vi "RT_Controller.vi"() -> ()   [LabVIEW 2017]
doc: "RT Controller with the coordinate transformation implemented, and with DSA!\n\nfor controlling FPGA controller with feedback linearization"
uses:
  <vilib>/rvi/interface/nirviReadWriteControl/nirviReadWriteControl.xnode
  <vilib>/Platform/TimedLoop/XDataNode/XDataNode.xnode
  <vilib>/Platform/TimedLoop/XDataNode/nitl_modes.ctl
  <vilib>/Platform/TimedLoop/XDataNode/XDNodeRunTimeDep.lvlib
  <vilib>/Platform/TimedLoop/XDataNode/wakeup.ctl
  <vilib>/Platform/TimedLoop/XDataNode/timing_clust.ctl
  Components/Timing/Timing.lvlib
  <vilib>/rvi/interface/nirviOpenFPGA/nirviOpenFPGA.xnode
  <vilib>/NI/STM/NI STM.lvlib
  <vilib>/NI/STM/SubVIs/MetaDataElement.ctl
  <vilib>/rvi/interface/nirviCloseFPGA/nirviCloseFPGA.xnode
  Components/DSA/DSA.lvlib
  <vilib>/Analysis/NI_AALPro.lvlib
  <vilib>/NI/STM/TCP/Write Message (TCP).vi
  TypeDefs/FPGA VI Reference.ctl
  <vilib>/ptbypt/NI_PtbyPt.lvlib
  TypeDefs/Ki.ctl
  <vilib>/NI/STM/TCP/Get Connection Reference (TCP).vi
  <vilib>/NI/STM/TCP/Write Meta Data (TCP Ref).vi
  FPGA Bitfiles/flexlab_FPGATarget_Tbeam256MAMainVI_XFHOL9u-69o.lvbitx
  NiFpgaLv.dll
  <vilib>/Utility/error.llb/Error Cluster From Error Code.vi
  <vilib>/rvi/errors/niLvFpgaAdjustHostInterfaceError.vi
  <vilib>/FPGAPlugInAG/myRIO-1900/niLvFpga_Close_myRIO-1900.vi
  <vilib>/FPGAPlugInAG/myRIO-1900/niLvFpga_Open_myRIO-1900.vi
  Components/SignalGen/SignalGenParams_Cluster.ctl
  Components/SignalGen/SignalGen.lvlib
  TypeDefs/ChZero_Cluster.ctl
  TypeDefs/BendTwist_Ref_Cluster.ctl
  TypeDefs/Kp.ctl
  TypeDefs/RefChEnum.ctl
panel:
  in  "Timing":enum32{"RT Loop", "DSA Loop", "While Loop"}(tab)=enum."While Loop"
  out "Finished late?":dbl
  out "Loop rate [Hz]":dbl=2000.0 min=0.0 step=100.0 format="%.2p"
  out "Finished late?":dbl
  out "Loop rate [Hz]":dbl=2000.0 min=0.0 step=100.0 format="%.2p"
  out "Number of iterations":i32
  in  "Select Operation Mode":enum32{"Settings", "Closed Loop"}(tab)=enum."Closed Loop"
  in  "Reset Zero":bool
  in  "Set Measurement Zero":bool
  in  "ChZero_Cluster":T1={"Bend Zero [V]"=-2.668583393096924, "Twist Zero [V]"=-0.010879039764404297} {"Twist Zero [V]" step=0.1; "Bend Zero [V]" step=0.1}
  in  "Twist Lead":T3={"Twist Lead Num (a0,a1)"=[-0.144109583, 0.144363337, 120.0], "Twist Lead Den (b0,b1)"=[0.984133655, -1.983879901, 120.0]} {"Twist Lead Den (b0,b1)" format="%#_5e"; "Twist Lead Num (a0,a1)" format="%#_5e"}
  in  "Ref Ch.":T4
  in  "Ref_Cluster":T5 {"Twist_ref [V]" step=0.001; "Bend_ref [V]" min=0.0 step=0.005 format="%#.4f"}
  in  "Run \nController?":bool
  in  "Kp":T6=[25.0, 20.0, 100000.0] format="%#_6p"
  in  "Ki*Ts":T2=[0.00062, 0.00045, 120.0] format="%#_5e"
  in  "Reference offset":T7={"phase"=0.0, "amplitude"=0.0, "frequency"=0.0, "offset"=0.0, "Signal"=enum."DSA"} {"offset" format="%0.2f"; "frequency" format="%#.4f"; "amplitude" step=0.01 format="%#.4f"; "phase" format="%0.2f"}
  in  "Bend Lead":T8={"Bend Lead Num (a0,a1)"=[-0.408503893706518, 0.409017557515985, 120.0], "Bend Lead Den (b0,b1)"=[0.968209299629241, -1.967695635819774, 120.0]} {"Bend Lead Den (b0,b1)" format="%#_5e"; "Bend Lead Num (a0,a1)" format="%#_5e"}
  in  "stop":bool
  in  "DSA":enum32{"DSA Controls", "DSA Plots"}(tab)
  in  "DSA Freq. Resp. Meas.":T9(ring)=enum."RR_bend"
  out "DSA\nRunning?":bool
  in  "Stop DSA":bool
  in  "Start DSA":bool
  in  "DSA excitation specs":T10={"Initial Freq. [Hz]"=5.0, "Final Freq. [Hz]"=990.0, "# pts. in interval"=30, "Samping Time [s]"=0.0005, "Amplitude"=0.01, "Offset [V]"=0.0, "Freq Units (F: rad/s, T: Hz)"=TRUE}
  in  "Cycle Specs":T11={"Cycles To \nSettle (M)"=5, "Cycles To \nCalculate (N)"=20}
  out "Phase Bode Plot":cluster{dbl[], dbl[]}(graph)
  out "Magnitude Bode Plot":cluster{dbl[], dbl[]}(graph)
  # "Run the PC_Controller.vi to enable running of main loop and transfer of data!"
  # "Make sure to select the correct Ref. Ch. \ne.g. RR_Bend requires \nRef. Ch. to be Bend"
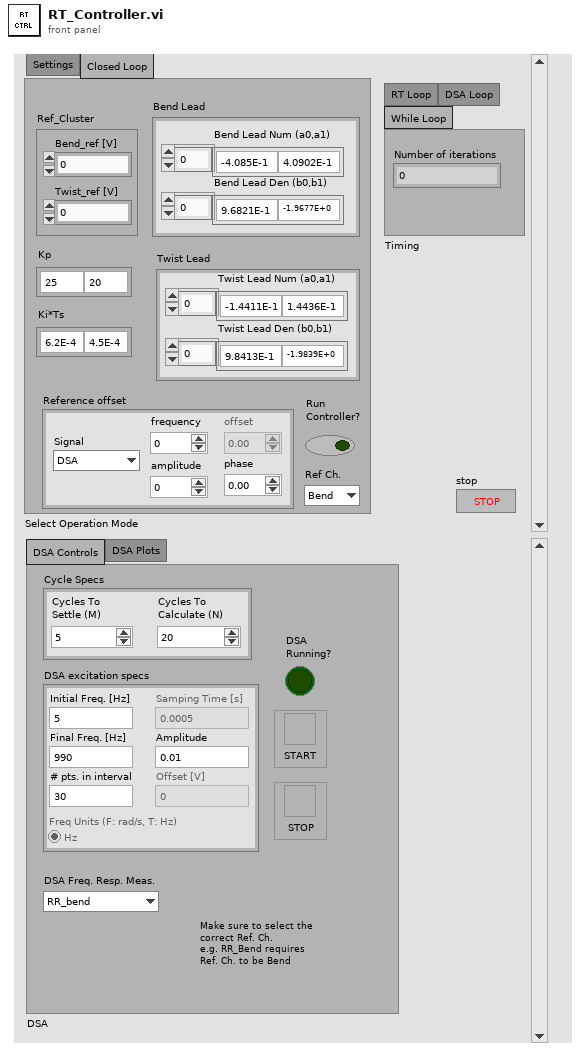
[diagram p1: front panel]
types:
  T1 = typedef "ChZero_Cluster.ctl" = cluster{"Bend Zero [V]":dbl, "Twist Zero [V]":dbl}
  T2 = typedef "Ki.ctl" = dbl[]
  T3 = cluster{"Twist Lead Num (a0,a1)":T2, "Twist Lead Den (b0,b1)":T2}
  T4 = typedef "RefChEnum.ctl" = enum16{"Bend", "Twist"}
  T5 = typedef "BendTwist_Ref_Cluster.ctl" = cluster{"Bend_ref [V]":dbl, "Twist_ref [V]":dbl}
  T6 = typedef "Kp.ctl" = dbl[]
  T7 = typedef "SignalGen.lvlib/SignalGenParams_Cluster.ctl" = cluster{"phase":dbl, "amplitude":dbl, "frequency":dbl, "offset":dbl, "Signal":enum16{"DC", "Sine", "Square", "Triangle", "Sawtooth", "DSA"}}
  T8 = cluster{"Bend Lead Num (a0,a1)":T2, "Bend Lead Den (b0,b1)":T2}
  T9 = enum16{"Plant_bend", "Plant_twist", "RR_bend", "RR_twist", "Ctrl_bend", "Ctrl_twist"}
  T10 = cluster{"Initial Freq. [Hz]":dbl, "Final Freq. [Hz]":dbl, "# pts. in interval":i16, "Samping Time [s]":dbl, "Amplitude":dbl, "Offset [V]":dbl, "Freq Units (F: rad/s, T: Hz)":bool}
  T11 = cluster{"Cycles To \nSettle (M)":i16, "Cycles To \nCalculate (N)":i16}
  T12 = typedef "NI STM.lvlib/MetaDataElement.ctl" = string
  T13 = typedef "FPGA VI Reference.ctl" = refnum<k20>
  T14 = typedef "NI STM.lvlib/TCP Connection Info.ctl" = cluster{"connection ID":refnum<k5>, "meta data":T12[]}
  T15 = typedef "XDNodeRunTimeDep.lvlib/timing_clust.ctl" = cluster{"Expected End [f-1]":u64, "Actual End [f-1]":u64, "Finished Late? [f-1]":bool, "Expected End [i-1]":u64, "Actual End [i-1]":u64, "Finished Late? [i-1]":bool, "Expected Start [i]":u64, "Actual Start [i]":u64, "Expected Start [f]":u64, "Actual Start [f]":u64, "Source Name":string, "Structure Name":string, "Period":i64, "Deadline":i64, "Offset":i64, "Start":i64, "Priority":i32, "Timeout":i32, "Mode":T16, "Wakeup Reason":T17, "Error":errorcluster, "Source Type":string, "Secondary Source Type":string, "Global End Time":u64, "Global Start Time":u64, "Frame Duration":u64, "Iteration Duration":u64, "Assigned CPU":i32, "I/O Scan Engine Mode":u32}
  T16 = typedef "XDNodeRunTimeDep.lvlib/nitl_modes.ctl" = enum32{"No Change", "Process missed periods, maintain original phase", "Discard missed periods, maintain original phase", "Process missed periods, ignore original phase", "Discard missed periods, ignore original phase"}
  T17 = typedef "XDNodeRunTimeDep.lvlib/wakeup.ctl" = enum32{"Normal", "Aborted", "Asynchronous wakeup", "Timing source error", "Timed loop error", "Timeout"}
  T18 = cluster{"Bend":cluster{"Notch Num (a0,a1,a2)":T2, "Notch Den (b0,b1)":T2}, "Twist":cluster{"Notch Num (a0,a1,a2)":T2, "Notch Den (b0,b1)":T2}}
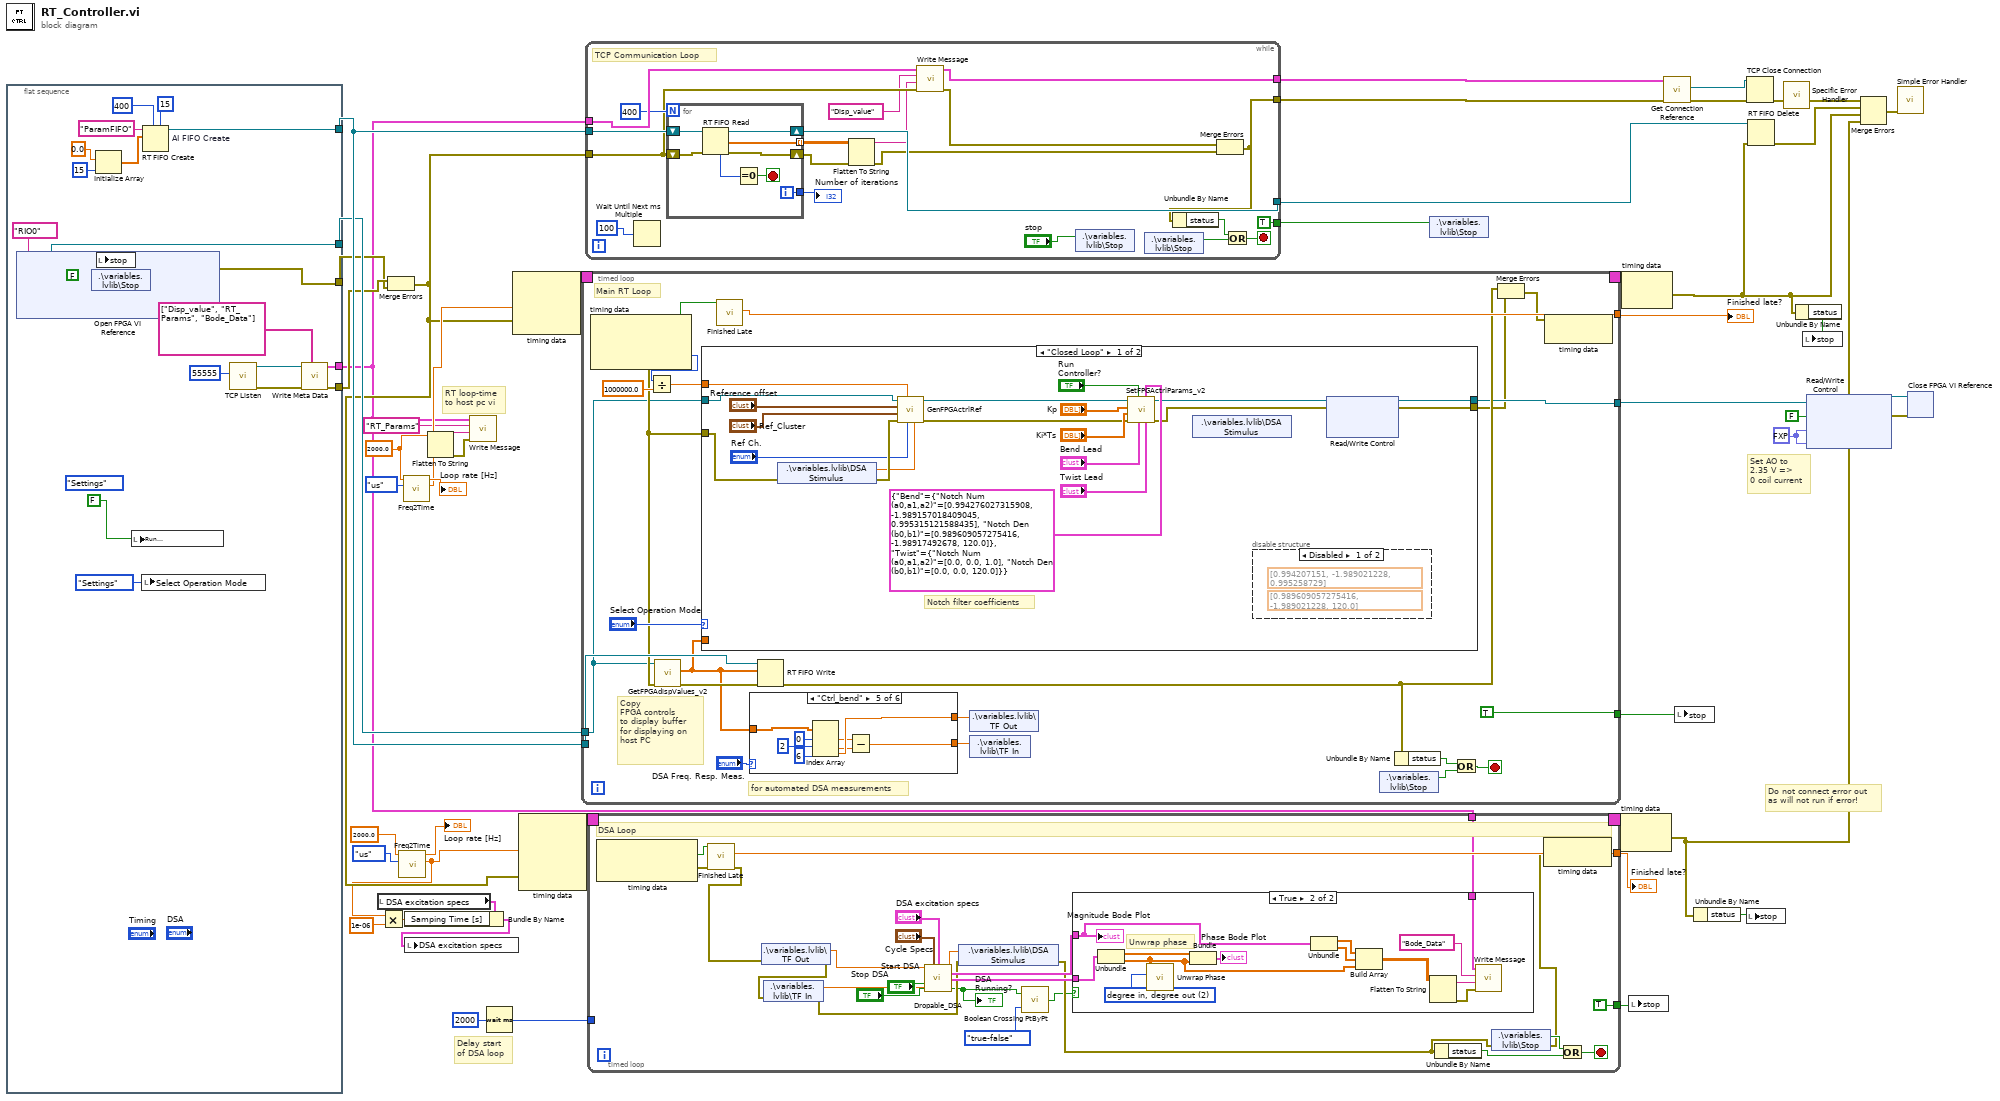
[diagram p0: block diagram]
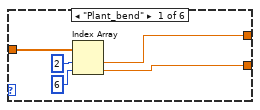
[diagram p2: hidden frame]
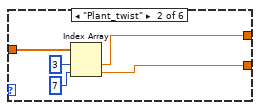
[diagram p3: hidden frame]
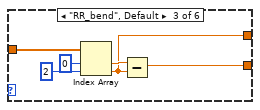
[diagram p4: hidden frame]
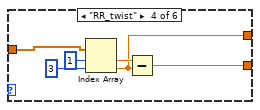
[diagram p5: hidden frame]
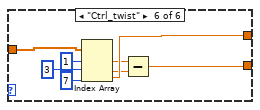
[diagram p6: hidden frame]
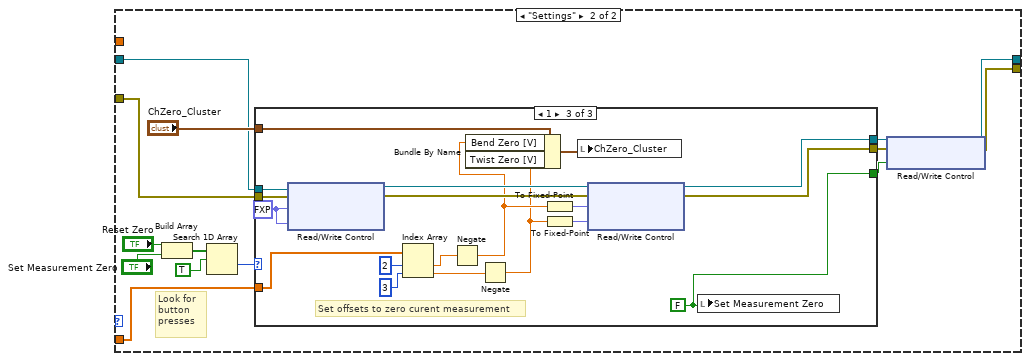
[diagram p8: hidden frame]
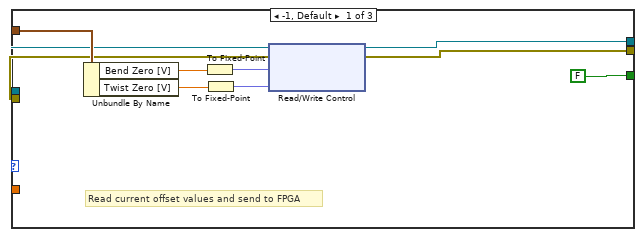
[diagram p9: hidden frame]
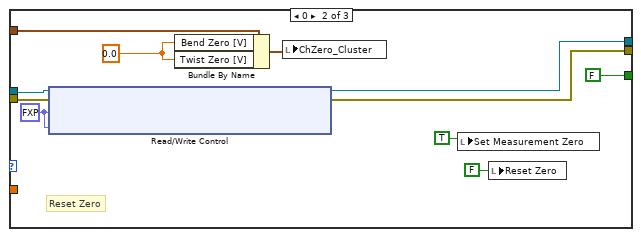
[diagram p10: hidden frame]
diagram:
  w1 = fxp<+,25,3> 0.0 ("AO Coil2 [V]")
  w9 = 2000.0 ("Period")
  # "Set AO to\n2.35 V => \n0 coil current"
  # "RT loop-time\nto host pc vi"
  # "Delay start\nof DSA loop"
  # "Do not connect error out\nas will not run if error!"
  n1 = flat-sequence {
    tunnel: [w68] -> w31
    tunnel: [w63] -> w3
    tunnel: [w62] -> w32
    tunnel: [w61] -> w40
    tunnel: [w59] -> w38
    frame #0 {
      (unwired) enum32{"Settings", "Open Loop", "Closed Loop"}."Settings" ("Select Operation Mode")
      w69 = FALSE ("Stop")
      n2 = xnode "Open FPGA VI Reference"("resource name"=tag "RIO0") -> ("FPGA VI Reference Out"=w59:T13, "error out"=w70:errorcluster)  [unwired: 1 in]
      n3 = shared-variable ".\\variables.lvlib\\Stop"(w69, error in=w70) -> (error out=w68:errorcluster)
      n4 = Initialize Array(0.0 ("element"), 15 ("dimension size")) -> (w55:dbl[])
      n5 = local write "stop"(w69) -> ()
      n6 = local write "Run \nController?"(FALSE ("Open Loop-Z?")) -> ()
      n7 = local write "Select Operation Mode"(enum32{"Settings", "Closed Loop"}."Settings" ("Select Operation Mode")) -> ()
      n8 = RT FIFO Create "AI FIFO Create"(0:"ParamFIFO" ("name (unnamed)"), 1:w55, 4:u32 400 ("size (10)"), 6:u32 15 ("elements in array (1)")) -> (8:w61:refnum<k33>)  [unwired: 4 in, 2 out]
      n9 = call <vilib>:"TCP Listen.vi"("port"=u16 55555) -> ("error out"=w66:errorcluster, "connection ID"=w65:refnum<k5>)  [unwired: 6 in, 3 out]
      n10 = call-poly <vilib>:"Write Meta Data.vi"("meta data"=T12[] ["Disp_value", "RT_Params", "Bode_Data"], "error in"=w66, "connection ID"=w65) -> ("error out"=w62:errorcluster, "connection info out"=w63:T14)  [unwired: 7 in]
    }
  }
  n11 = local read "DSA excitation specs"() -> (w6:T10)
  n12 = Merge Errors(w32, w31) -> (w13:errorcluster)
  n13 = call "Freq2Time.vi"("Int. Time Unit"=enum16{"sec", "us", "ms"}."us", "Sample rate (Hz)"=2000.0 ("Period")) -> ("Int.  time [unit]"=w7:dbl, "New Sample rate (Hz)"=→"Loop rate [Hz]":dbl)  [unwired: 7 in, 1 out]
  n14 = Multiply(x=w7, y=1e-06) -> (x*y=w5:dbl)
  n15 = call "Freq2Time.vi"("Int. Time Unit"=enum16{"sec", "us", "ms"}."us", "Sample rate (Hz)"=w9) -> ("Int.  time [unit]"=w27:dbl, "New Sample rate (Hz)"=→"Loop rate [Hz]":dbl)  [unwired: 7 in, 1 out]
  n16 = Bundle By Name(cluster=w6, "Samping Time [s]"=w5) -> (w4:T10)
  n17 = local write "DSA excitation specs"(w4) -> ()
  n18 = Flatten To String(anything=w9) -> (data string=w10:string, error out=w11:errorcluster)  [unwired: 3 in, 1 out]
  n19 = call-poly <vilib>:"Write Message.vi"("error in"=w11, "data"=w10, "name"="RT_Params", "connection info in"=w3) -> ()  [unwired: 6 in, 2 out]
  n20 = Wait (ms)(milliseconds to wait=u32 2000) -> (millisecond timer value=w14:u32)
  n21 = node-c288(w27, w13) -> (w50:T15)  [unwired: 1 in]
  n22 = node-c288(w7, w13) -> (w26:T15)  [unwired: 2 in]
  n23 = timed-loop "Timed Loop" {
    timing: w50 -> [_]
    timing-out: [_] -> w49
    tunnel: [w91] -> w48
    tunnel: w40 -> [w79]
    tunnel: w38 -> [w71]
    tunnel: [w84] -> w36
    tunnel: [TRUE ("Stop")] -> w16
    stop <- w90 stop-if-true
    # "Main RT Loop"
    # "for automated DSA measurements"
    # "Copy \nFPGA controls\nto display buffer \nfor displaying on host PC"
    n24 = node-c288() -> (w75:errorcluster, w92:bool, w81:i64)  [unwired: 1 in]
    n25 = Divide(x=w81, y=1000000.0) -> (x/y=w80:dbl)
    n26 = call "GetFPGAdispValues_v2.vi"("error in (no error)"=w75, "FPGA VI Reference In"=w71) -> ("error out"=w74:errorcluster, "State variables"=w73:dbl[])  [unwired: 7 in, 1 out]
    n27 = case shown="\"Closed Loop\"" "Select Operation Mode" {
      tunnel: w71 -> [w147 w170]
      tunnel: [w141 w160] -> w84
      tunnel: w75 -> [w153 w169]
      tunnel: [w139 w161] -> w83
      tunnel: w80 -> [w154 _]
      tunnel: w73 -> [_ w159]
      frame "Closed Loop" {
        # "Notch filter coefficients"
        # "Notch filter"
        n28 = shared-variable ".\\variables.lvlib\\DSA Stimulus"(error in=w153) -> (w138:dbl, error out=w152:errorcluster)
        n29 = call "GenFPGActrlRef.vi"("DSA excitation"=w138, "Ref Ch."="Ref Ch.", "Current Time [s]"=w154, "error in (no error)"=w152, "Z,ThX,ThY Ref_Cluster"="Ref_Cluster", "Reference Offset"="Reference offset", "FPGA Interface"=w147) -> ("error out"=w146:errorcluster, "FPGA VI Reference Out"=w151:T13)  [unwired: 2 in, 1 out]
        n30 = call "SetFPGActrlParams_v2.vi"("Twist Lead"="Twist Lead", "Notch"=T18 {"Bend"={"Notch Num (a0,a1,a2)"=[0.994276027315908, -1.989157018409045, 0.995315121588435], "Notch Den (b0,b1)"=[0.989609057275416, -1.98917492678, 120.0]}, "Twist"={"Notch Num (a0,a1,a2)"=[0.0, 0.0, 1.0], "Notch Den (b0,b1)"=[0.0, 0.0, 120.0]}}, "Bend Lead"="Bend Lead", "Run Controller?"="Run \nController?", "error in (no error)"=w146, "Ki*Ts"="Ki*Ts", "Kp"="Kp", "FPGA VI Reference In"=w151) -> ("error out"=w140:errorcluster, "FPGA VI Reference Out"=w142:T13)  [unwired: 2 in]
        n31 = shared-variable ".\\variables.lvlib\\DSA Stimulus"() -> ()  [unwired: 1 in, 2 out]
        n32 = disable-structure shown="Disabled" {
          frame Disabled {
            (unwired) T2 [0.989609057275416, -1.989021228, 120.0] ("Notch Den (b0,b1)")
            (unwired) T2 [0.994207151, -1.989021228, 0.995258729] ("Notch Num (a0,a1,a2)")
          }
          frame Enabled {
          }
        }
        n33 = xnode "Read/Write Control"("FPGA VI Reference In"=w142, "error in"=w140) -> ("FPGA VI Reference Out"=w141:T13, "error out"=w139:errorcluster)  [unwired: 2 in]
      }
      frame "Settings" {
        # "Look for \nbutton\npresses"
        n34 = Build Array "Build Array"("Reset Zero", "Set Measurement Zero") -> (w168:bool[])
        n35 = Search 1D Array(1D array=w168, element=TRUE) -> (index of element=w164:i32)  [unwired: 1 in]
        n36 = case shown="1" w164 {
          tunnel: "ChZero_Cluster" -> [w181 w190 w210]
          tunnel: w170 -> [w179 w192 w205]
          tunnel: [w178 w188 w209] -> w163
          tunnel: w169 -> [w180 w191 w207]
          tunnel: [w177 w187 w208] -> w162
          tunnel: w159 -> [_ _ w203]
          tunnel: [FALSE ("Run Controller?") FALSE ("Run Controller?") w199] -> w158
          frame -1, Default {
            # "Read current offset values and send to FPGA"
            n37 = Unbundle By Name(w181) -> ("Bend Zero [V]"=w176:dbl, "Twist Zero [V]"=w175:dbl)
            n38 = To Fixed-Point(number=w176) -> (fixed-point=w174:fxp<+/-,26,4>)  [unwired: 1 in]
            n39 = To Fixed-Point(number=w175) -> (fixed-point=w173:fxp<+/-,26,4>)  [unwired: 1 in]
            n40 = xnode "Read/Write Control"("FPGA VI Reference In"=w179, "error in"=w180, "Bend offset [V]"=w174, "Twist offset [V]"=w173) -> ("FPGA VI Reference Out"=w178:T13, "error out"=w177:errorcluster)
          }
          frame 0 {
            w189 = 0.0 ("Ch0_Zero [mm]")
            w182 = fxp<+/-,26,4> 0.0 ("Ch0 zero [mm]")
            # "Reset Zero"
            n41 = xnode "Read/Write Control"("FPGA VI Reference In"=w192, "error in"=w191, "Bend offset [V]"=w182, "Twist offset [V]"=w182) -> ("FPGA VI Reference Out"=w188:T13, "error out"=w187:errorcluster)
            n42 = Bundle By Name(cluster=w190, "Bend Zero [V]"=w189, "Twist Zero [V]"=w189) -> (w186:T1)
            n43 = local write "ChZero_Cluster"(w186) -> ()
            n44 = local write "Set Measurement Zero"(TRUE ("Set Measurement Zero")) -> ()
            n45 = local write "Reset Zero"(FALSE ("Reset Zero")) -> ()
          }
          frame 1 {
            w200 = fxp<+/-,26,4> 0.0 ("Ch0 zero [mm]")
            w199 = FALSE ("Set Zero")
            # "Set offsets to zero curent measurement"
            n46 = xnode "Read/Write Control"("FPGA VI Reference In"=w205, "error in"=w207, "Bend offset [V]"=w200, "Twist offset [V]"=w200) -> ("FPGA VI Reference Out"=w204:T13, "error out"=w206:errorcluster)
            n47 = Index Array(array=w203, index #1=2 ("index"), index #2=3 ("index")) -> (element #1=w198:dbl, element #2=w197:dbl)
            n48 = Negate(x=w198) -> (-x=w194:dbl)
            n49 = Negate(x=w197) -> (-x=w193:dbl)
            n50 = Bundle By Name(cluster=w210, "Bend Zero [V]"=w194, "Twist Zero [V]"=w193) -> (w211:T1)
            n51 = To Fixed-Point(number=w194) -> (fixed-point=w196:fxp<+/-,26,4>)  [unwired: 1 in]
            n52 = To Fixed-Point(number=w193) -> (fixed-point=w195:fxp<+/-,26,4>)  [unwired: 1 in]
            n53 = local write "ChZero_Cluster"(w211) -> ()
            n54 = xnode "Read/Write Control"("FPGA VI Reference In"=w204, "error in"=w206, "Bend offset [V]"=w196, "Twist offset [V]"=w195) -> ("FPGA VI Reference Out"=w209:T13, "error out"=w208:errorcluster)
            n55 = local write "Set Measurement Zero"(w199) -> ()
          }
        }
        n56 = xnode "Read/Write Control"("FPGA VI Reference In"=w163, "error in"=w162, "Run controller?"=w158) -> ("FPGA VI Reference Out"=w160:T13, "error out"=w161:errorcluster)
      }
    }
    n57 = call "Finished Late.vi"("Finished \nLate?"=w92) -> ("# Finished\nLate counter"=w91:dbl)  [unwired: 8 in, 2 out]
    n58 = case shown="\"Ctrl_bend\"" "DSA Freq. Resp. Meas." {
      tunnel: [w93 w98 w106 w112 w118 w126] -> w77
      tunnel: [w95 w100 w103 w109 w117 w125] -> w72
      tunnel: w73 -> [w94 w99 w104 w111 w120 w128]
      frame "Plant_bend" {
        n59 = Index Array(array=w94, index #1=2 ("index"), index #2=6 ("index")) -> (element #1=w95:dbl, element #2=w93:dbl)
      }
      frame "Plant_twist" {
        n60 = Index Array(array=w99, index #1=3 ("index"), index #2=7 ("index")) -> (element #1=w100:dbl, element #2=w98:dbl)
      }
      frame "RR_bend", Default {
        n61 = Index Array(array=w104, index #1=0 ("index"), index #2=2 ("index")) -> (element #1=w105:dbl, element #2=w103:dbl)
        n62 = Subtract(x=w105, y=w103) -> (x-y=w106:dbl)
      }
      frame "RR_twist" {
        n63 = Index Array(array=w111, index #1=1 ("index"), index #2=3 ("index")) -> (element #1=w110:dbl, element #2=w109:dbl)
        n64 = Subtract(x=w110, y=w109) -> (x-y=w112:dbl)
      }
      frame "Ctrl_bend" {
        n65 = Index Array(array=w120, index #1=0 ("index"), index #2=2 ("index"), index #3=6 ("index")) -> (element #1=w116:dbl, element #2=w115:dbl, element #3=w117:dbl)
        n66 = Subtract(x=w116, y=w115) -> (x-y=w118:dbl)
      }
      frame "Ctrl_twist" {
        n67 = Index Array(array=w128, index #1=1 ("index"), index #2=3 ("index"), index #3=7 ("index")) -> (element #1=w124:dbl, element #2=w123:dbl, element #3=w125:dbl)
        n68 = Subtract(x=w124, y=w123) -> (x-y=w126:dbl)
      }
    }
    n69 = RT FIFO Write(0:w79, 1:w73, 3:w74) -> (11:w87:errorcluster)  [unwired: 2 in, 3 out]
    n70 = shared-variable ".\\variables.lvlib\\TF Out"(w72) -> ()  [unwired: 1 in, 1 out]
    n71 = shared-variable ".\\variables.lvlib\\TF In"(w77) -> ()  [unwired: 1 in, 1 out]
    n72 = shared-variable ".\\variables.lvlib\\Stop"() -> (w89:bool)  [unwired: 1 in, 1 out]
    n73 = Unbundle By Name(w87) -> ("status"=w88:bool)
    n74 = Or(x=w88, y=w89) -> (x .or. y?=w90:bool)
    n75 = Merge Errors(w87, w83) -> (w86:errorcluster)
    n76 = node-c288(w86) -> ()  [unwired: 1 out]
  }
  "Finished late?" <- w48
  n77 = while {
    tunnel: w3 -> [w230]
    tunnel: w13 -> [w219]
    tunnel: w40 -> [w225]
    tunnel: [w223] -> w42
    tunnel: [w215] -> w37
    tunnel: [w214] -> w34
    tunnel: [TRUE ("Stop")] -> w30
    stop <- w227 stop-if-true
    # "TCP Communication Loop"
    n78 = Wait Until Next ms Multiple(millisecond multiple=u32 100) -> ()  [unwired: 1 out]
    n79 = for {
      N: 400 -> [_]
      shift-right: [w236] -> w223
      shift-left: w225 -> [w239]
      shift-right: [w238] -> w224
      shift-left: w219 -> [w237]
      tunnel: [w233] -> w222
      tunnel: [w232] -> w218 mode=indexing
      i -> [w233]
      stop <- w234 stop-if-true
      n80 = RT FIFO Read(0:w239, 3:w237) -> (7:w235:u32, 8:w236:refnum<k33>, 9:w232:dbl[], 11:w238:errorcluster)  [unwired: 2 in, 1 out]
      n81 = Equal To 0?(x=w235) -> (x = 0?=w234:bool)
    }
    "Number of iterations" <- w222
    n82 = Flatten To String(anything=w218, error in (no error)=w224) -> (data string=w216:string, error out=w220:errorcluster)  [unwired: 2 in, 1 out]
    n83 = call-poly <vilib>:"Write Message.vi"("error in"=w219, "data"=w216, "name"="Disp_value", "connection info in"=w230) -> ("error out"=w213:errorcluster, "connection info out"=w214:T14)  [unwired: 6 in]
    n84 = shared-variable ".\\variables.lvlib\\Stop"("stop") -> ()  [unwired: 1 in, 1 out]
    n85 = shared-variable ".\\variables.lvlib\\Stop"() -> (w229:bool)  [unwired: 1 in, 1 out]
    n86 = Merge Errors(w213, w220) -> (w215:errorcluster)
    n87 = Unbundle By Name(w215) -> ("status"=w228:bool)
    n88 = Or(x=w228, y=w229) -> (x .or. y?=w227:bool)
  }
  n89 = timed-loop "DSA" {
    timing: w26 -> [_]
    timing-out: [_] -> w25
    tunnel: [TRUE ("Stop")] -> w17
    tunnel: [w255] -> w23
    tunnel: w14 -> [_]
    tunnel: w3 -> [w243]
    stop <- w251 stop-if-true
    # "DSA Loop"
    n90 = node-c288() -> (w256:bool, w248:errorcluster)  [unwired: 1 in]
    n91 = call "Finished Late.vi"("error in (no error)"=w248, "Finished \nLate?"=w256) -> ("error out"=w247:errorcluster, "# Finished\nLate counter"=w255:dbl)  [unwired: 7 in, 1 out]
    n92 = shared-variable ".\\variables.lvlib\\TF Out"(error in=w247) -> (w253:dbl, error out=w250:errorcluster)
    n93 = shared-variable ".\\variables.lvlib\\TF In"(error in=w250) -> (w252:dbl, error out=w249:errorcluster)
    n94 = call "Dropable_DSA.vi"("TF Out (CH B)"=w253, "Cycle Specs"="Cycle Specs", "Excitation Specs"="DSA excitation specs", "TF In (CH A)"=w252, "START"="Start DSA", "STOP"="Stop DSA") -> ("Disturbance"=w254:dbl, "Bode Magnitude"=w260:cluster{dbl[], dbl[]}, "Bode Phase"=w259:cluster{dbl[], dbl[]}, "Running"=w241:bool)  [unwired: 4 in, 2 out]
    "DSA\nRunning?" <- w241
    n95 = shared-variable ".\\variables.lvlib\\DSA Stimulus"(w254, error in=w249) -> (error out=w246:errorcluster)
    n96 = call <vilib>:"Boolean Crossing PtByPt.vi"("direction"=enum16{"either", "false-true", "true-false"}."true-false", "input"=w241) -> ("crossing"=w240:bool)  [unwired: 1 in]
    n97 = case shown="True" w240 {
      tunnel: w260 -> [_ w267]
      tunnel: w259 -> [_ w277]
      tunnel: w243 -> [_ w266]
      frame False {
      }
      frame True {
        w275 = 2 items=["radian in, radian out", "radian in, degree out", "degree in, degree out", "degree in, radian out"] ("phase unit")
        # "Unwrap phase"
        n98 = Unbundle(w277) -> (w276:dbl[], w265:dbl[])
        n99 = call <vilib>:"Unwrap Phase.vi"("phase unit"=w275, "Phase"=w265) -> ()  [unwired: 8 in, 2 out]
        n100 = Bundle(w276, w265) -> (→"Phase Bode Plot":cluster{dbl[], dbl[]})  [unwired: 1 in]
        n101 = Unbundle(w267) -> (w273:dbl[], w272:dbl[])
        n102 = Build Array(w273, w272, w265) -> (w271:dbl[][])
        n103 = Flatten To String(anything=w271) -> (data string=w269:string, error out=w270:errorcluster)  [unwired: 3 in, 1 out]
        n104 = call-poly <vilib>:"Write Message.vi"("error in"=w270, "data"=w269, "name"="Bode_Data", "connection info in"=w266) -> ()  [unwired: 6 in, 2 out]
        "Magnitude Bode Plot" <- w267
      }
    }
    n105 = Unbundle By Name(w246) -> ("status"=w257:bool)
    n106 = shared-variable ".\\variables.lvlib\\Stop"(error in=w246) -> (w264:bool, error out=w245:errorcluster)
    n107 = node-c288(w245) -> ()  [unwired: 1 out]
    n108 = Or(x=w264, y=w257) -> (x .or. y?=w251:bool)
  }
  "Finished late?" <- w23
  n109 = shared-variable ".\\variables.lvlib\\Stop"(w30) -> ()  [unwired: 1 in, 1 out]
  n110 = node-c288(w25) -> (w24:errorcluster)
  n111 = node-c288(w49) -> (w20:errorcluster)
  n112 = local write "stop"(w17) -> ()
  n113 = call-poly <vilib>:"Get Connection Reference.vi"("error in"=w37, "connection info in"=w34) -> ("error out"=w46:errorcluster, "connection ID out"=w45:refnum<k5>)  [unwired: 7 in, 1 out]
  n114 = local write "stop"(w16) -> ()
  n115 = Unbundle By Name(w24) -> ("status"=w18:bool)
  n116 = local write "stop"(w18) -> ()
  n117 = TCP Close Connection(connection ID=w45, error in (no error)=w46) -> (error out=w44:errorcluster)  [unwired: 1 in, 1 out]
  n118 = RT FIFO Delete(0:w42, 3:w20) -> (11:w41:errorcluster)  [unwired: 1 in]
  n119 = call "Specific Error Handler"("Error to Check"=w44) -> ("error out"=w33:errorcluster)  [unwired: 11 in, 3 out]
  n120 = Unbundle By Name(w20) -> ("status"=w19:bool)
  n121 = local write "stop"(w19) -> ()
  n122 = xnode "Read/Write Control"("FPGA VI Reference In"=w36, "Run controller?"=FALSE ("AO enabled?"), "U_twist [V]"=w1, "U_bend [V]"=w1) -> ("FPGA VI Reference Out"=w29:T13, "error out"=w28:errorcluster)  [unwired: 1 in]
  n123 = Merge Errors(w33, w41, w20, w24) -> (w43:errorcluster)
  n124 = call <vilib>:"Simple Error Handler.vi"("error in (no error)"=w43) -> ()  [unwired: 4 in, 5 out]
  n125 = xnode "Close FPGA VI Reference"("FPGA VI Reference In"=w29, "error in"=w28) -> ()  [unwired: 1 out]
